vi "__Convert Cloud List data for Display.vi"(10 "Folders":string[](array[string]), 11 "Objects":T1[](array[typedef])) -> (2 "Symbols":i32[](array[numeric]), 3 "List data":string[][](array[string]))   [LabVIEW 2011]
doc: "Parses the data received when listing a cloud path to the format that is required to display it on the multicolumn listbox."
uses:
  __Cloud Object Info type.ctl
  vi.lib/National Instruments/LabVIEW Interface for Amazon S3/Typedefs/AMZ_S3_Storage Class.ctl
  vi.lib/National Instruments/LabVIEW Interface for Amazon S3/LV Interface for Amazon S3.lvlib
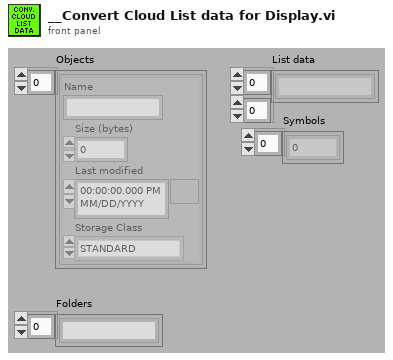
[diagram p1: front panel]
types:
  T1 = typedef "__Cloud Object Info type.ctl" = cluster{"Name":string, "Size (bytes)":u64, "Last modified":timestamp, "Storage Class":T2}
  T2 = typedef "LV Interface for Amazon S3.lvlib/AMZ_S3_Storage Class.ctl" = enum16{"STANDARD", "REDUCED_REDUNDANCY"}
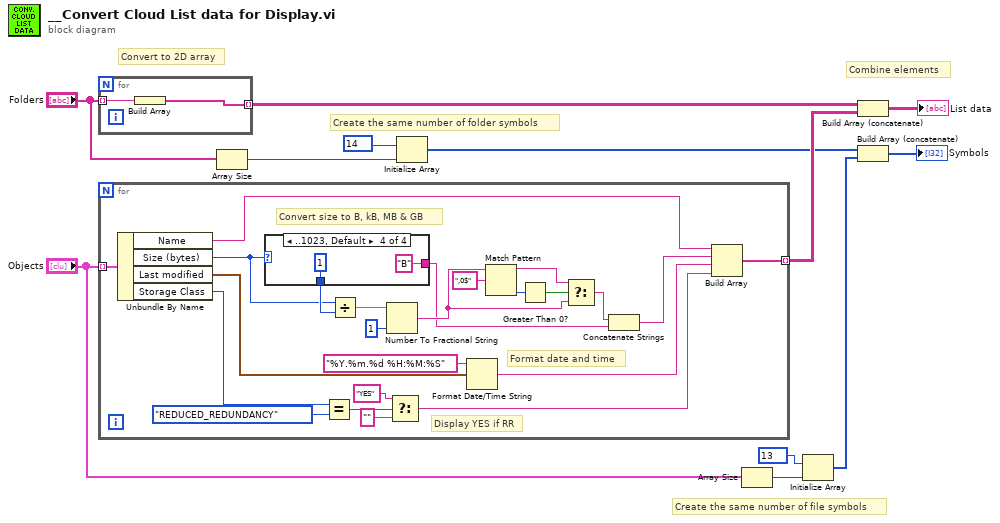
[diagram p0: block diagram]
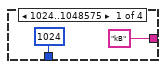
[diagram p2: hidden frame]
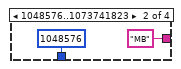
[diagram p3: hidden frame]
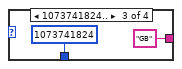
[diagram p4: hidden frame]
diagram:
  # "Combine elements"
  # "Create the same number of file symbols"
  # "Create the same number of folder symbols"
  # "Convert to 2D array"
  n1 = for {
    tunnel: "Folders" -> [w14] mode=indexing
    tunnel: [w13] -> w5 mode=indexing
    n2 = Build Array(w14) -> (w13:string[])
  }
  n3 = for {
    tunnel: "Objects" -> [w38] mode=indexing
    tunnel: [w15] -> w6 mode=indexing
    # "Convert size to B, kB, MB & GB"
    # "Format date and time"
    # "Display YES if RR"
    n4 = Unbundle By Name(w38) -> ("Name"=w24:string, "Size (bytes)"=w27:u64, "Last modified"=w25:timestamp, "Storage Class"=w21:T2)
    n5 = case shown="..1023, Default" w27 {
      tunnel: [u64 1024 ("size") u64 1048576 ("size") u64 1073741824 ("size") u64 1 ("size")] -> w29
      tunnel: ["kB" ("string") "MB" ("string") "GB" ("string") "B" ("string")] -> w30
      frame 1024..1048575 {
      }
      frame 1048576..1073741823 {
      }
      frame 1073741824.. {
      }
      frame ..1023, Default {
      }
    }
    n6 = Equal?(x=w21, y=AMZ_S3_Storage_Class."REDUCED_REDUNDANCY") -> (x = y?=w19:bool)
    n7 = Divide(x=w27, y=w29) -> (x/y=w28:dbl)
    n8 = Number To Fractional String(number=w28, precision (6)=i16 1) -> (F-format string=w36:string)  [unwired: 2 in]
    n9 = Select(t="YES" ("regular expression"), s=w19, f="") -> (s? t:f=w16:string)
    n10 = Format Date/Time String(time format string (%c)="%Y.%m.%d %H:%M:%S", seconds (now)=w25) -> (date/time string=w22:string)  [unwired: 1 in]
    n11 = Match Pattern(string=w36, regular expression=",0$") -> (before substring=w35:string, offset past match=w33:i32)  [unwired: 1 in, 2 out]
    n12 = Greater Than 0?(x=w33) -> (x > 0?=w34:bool)
    n13 = Select(t=w35, s=w34, f=w36) -> (s? t:f=w37:string)
    n14 = Concatenate Strings(w37, w30) -> (w23:string)
    n15 = Build Array(w24, w23, w22, w16) -> (w15:string[])
  }
  n16 = Array Size(array="Folders") -> (size(s)=w9:i32)
  n17 = Initialize Array(14, w9) -> (w4:i32[])
  n18 = Array Size(array="Objects") -> (size(s)=w11:i32)
  n19 = Initialize Array(13, w11) -> (w3:i32[])
  n20 = Build Array (concatenate)(w5, w6) -> (→"List data":string[][])
  n21 = Build Array (concatenate)(w4, w3) -> (→"Symbols":i32[])
